vi "SendArrayRowToLowLevel.vi"(8 "error in (no error)":errorcluster, 9 "all rows":i64[][](array[numeric]), 10 "Numeric":i32, 11 "Queue in":refnum<queue>) -> (0 "error out":errorcluster)   [LabVIEW 2017]
uses:
  LowLevel cluster.ctl
  LowLevelMsg.ctl
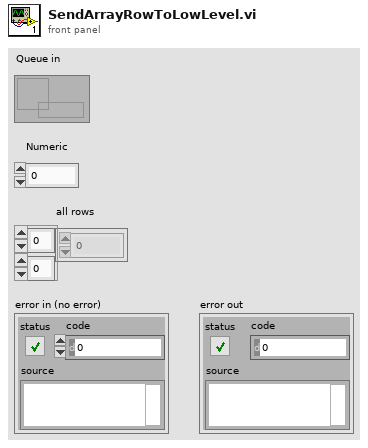
[diagram p1: front panel]
types:
  T1 = typedef "LowLevelMsg.ctl" = enum16{"ResetArduinoState", "Init", "Halt", "SetArduinoState", "RunStopSigGen", "Error"}
  T2 = typedef "LowLevel cluster.ctl" = cluster{"LowLevelMsg":T1, "LowLevel string":string}
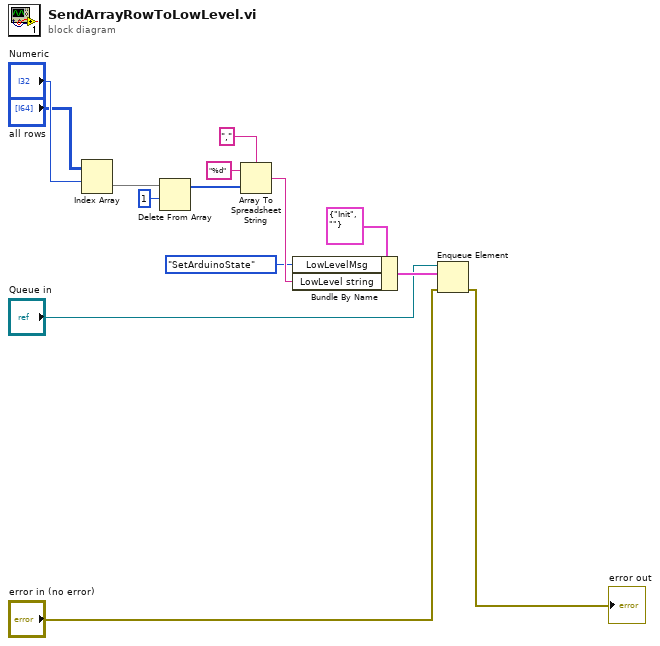
[diagram p0: block diagram]
diagram:
  n1 = Index Array(array="all rows", index (row)="Numeric") -> (element=w3:i64[])  [unwired: 1 in]
  n2 = Delete From Array(array=w3, length=1) -> (array with subset deleted=w5:i64[])  [unwired: 1 in, 1 out]
  n3 = Array To Spreadsheet String(delimiter (Tab)=",", array=w5, 3:"%d" ("format string")) -> (spreadsheet string=w11:string)
  n4 = Bundle By Name(cluster=T2 {"LowLevelMsg"=enum."Init", "LowLevel string"=""} ("element"), "LowLevelMsg"=LowLevelMsg."SetArduinoState", "LowLevel string"=w11) -> (w12:T2)
  n5 = Enqueue Element(queue="Queue in", element=w12, error in (no error)="error in (no error)") -> (error out=→"error out":errorcluster)  [unwired: 1 in, 2 out]
